vi "Find Broken VIs.vi"() -> ()   [LabVIEW 2016]
doc: "A wrapper engine for finding the list of broken VIs in a folder."
uses:
  <vilib>/Utility/error.llb/DialogType.ctl
  SLL Queued State Machine/Queue Driver/Create Queue.vi
  SLL Queued State Machine/Queue Driver/Enqueue an Item to Queue.vi
  SLL Queued State Machine/Queue Driver/Dequeue Queue.vi
  SLL Queued State Machine/Queue Driver/Enqueue N Items.vi
  SLL Queued State Machine/Queue Driver/Flush Queue.vi
  SLL Queued State Machine/Queue Driver/Release Queue.vi
  SLL Queued State Machine/SLL QSM.lvlib
  SLL Scripting/SLL Scripting.lvlib
panel:
  out "Number of VIs Broken":i32
  out "VIs Broken[]":path[](array[path])
  in  "Folder Path":path
  out "Status":string
  in  "Run":bool
  # "Find Broken VIs"
  # "Finds the list of broken VIs in a folder."
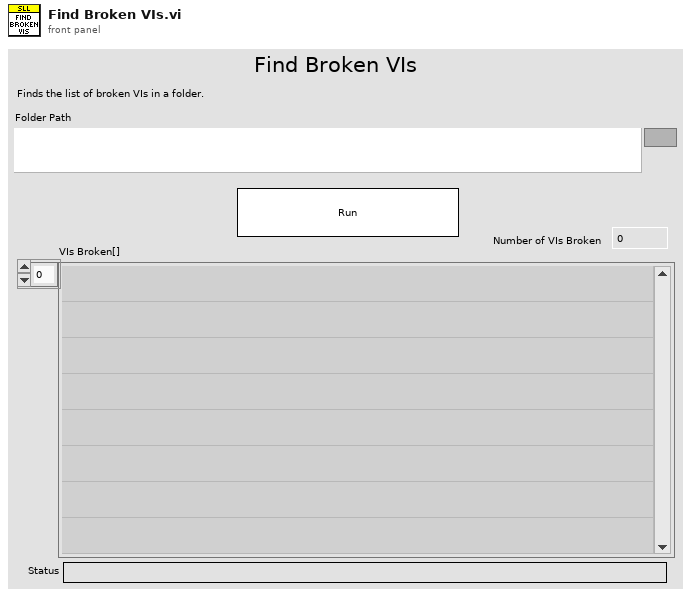
[diagram p1: front panel]
types:
  T1 = typedef "DialogType.ctl" = u16
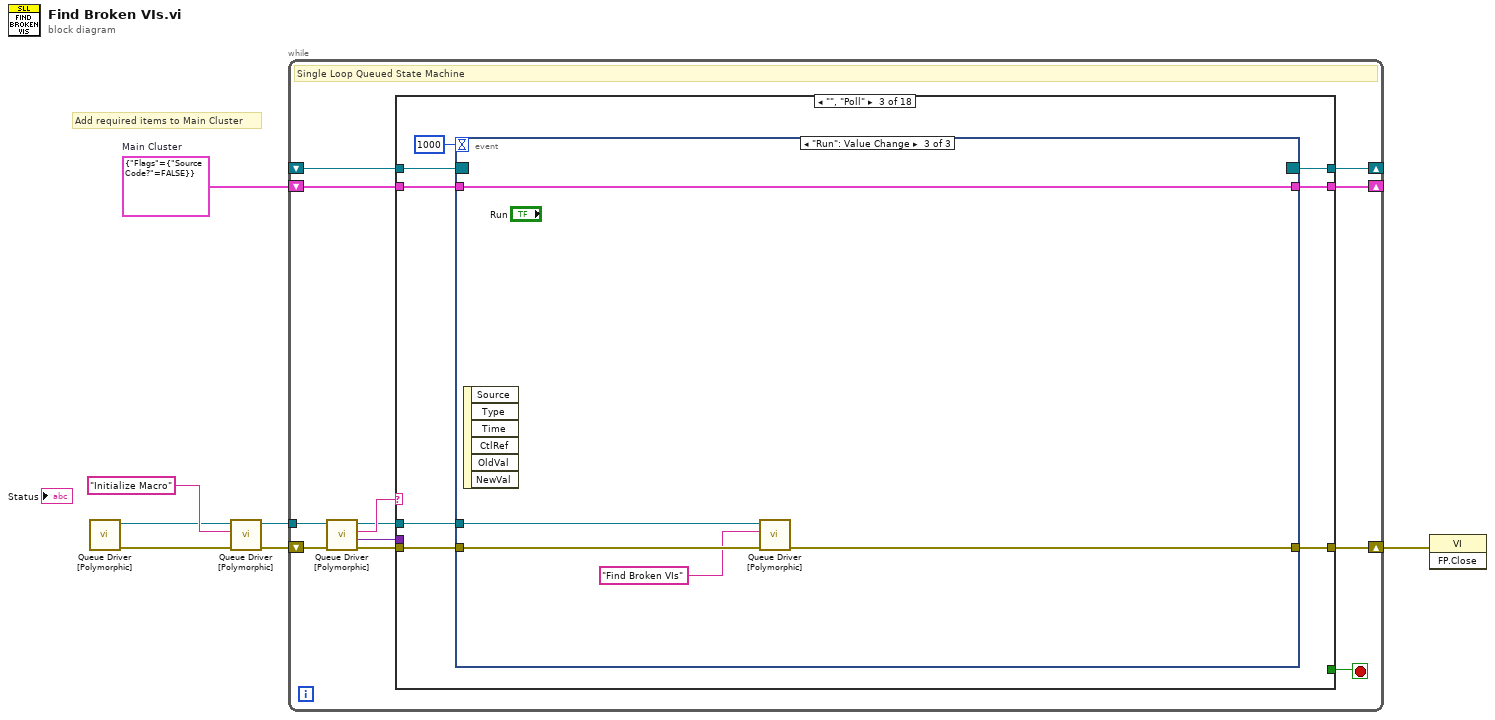
[diagram p0: block diagram]
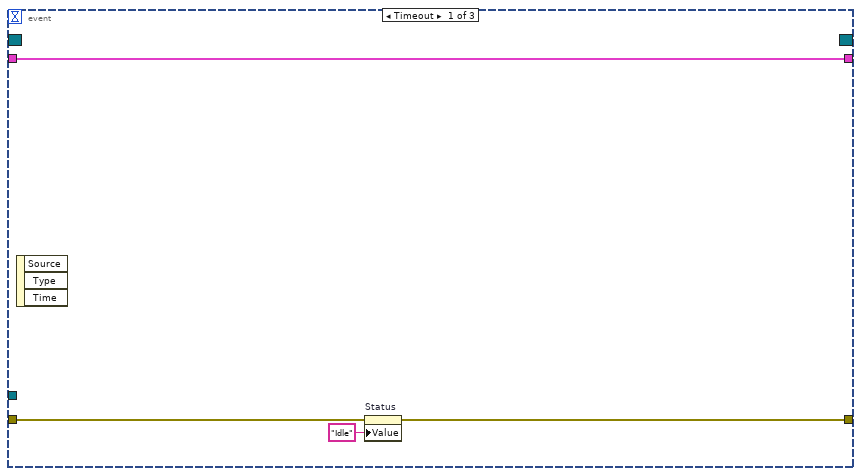
[diagram p4: hidden frame]
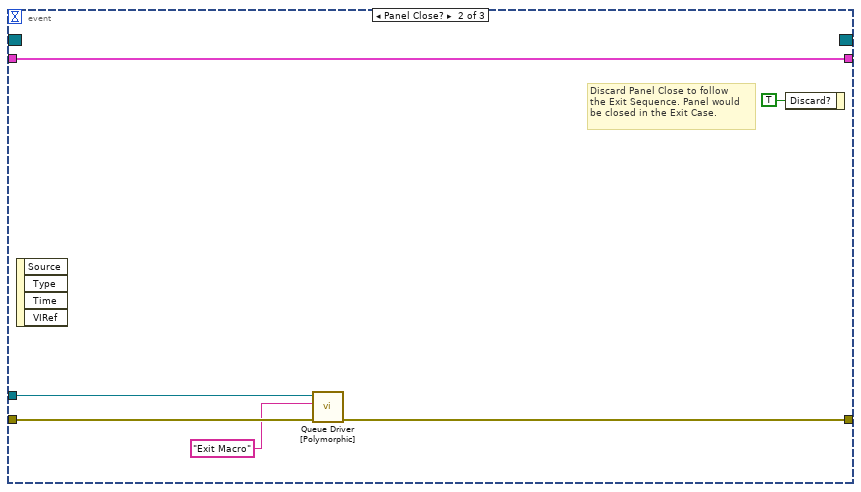
[diagram p5: hidden frame]
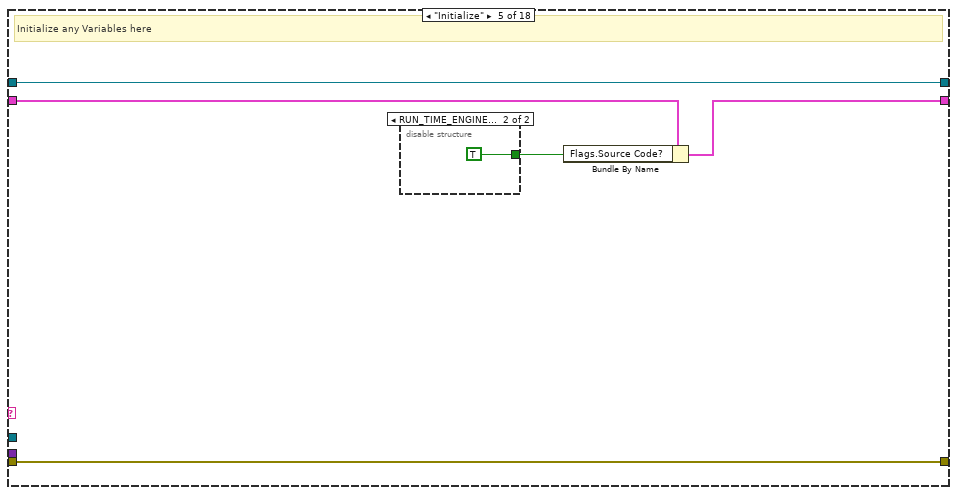
[diagram p7: hidden frame]
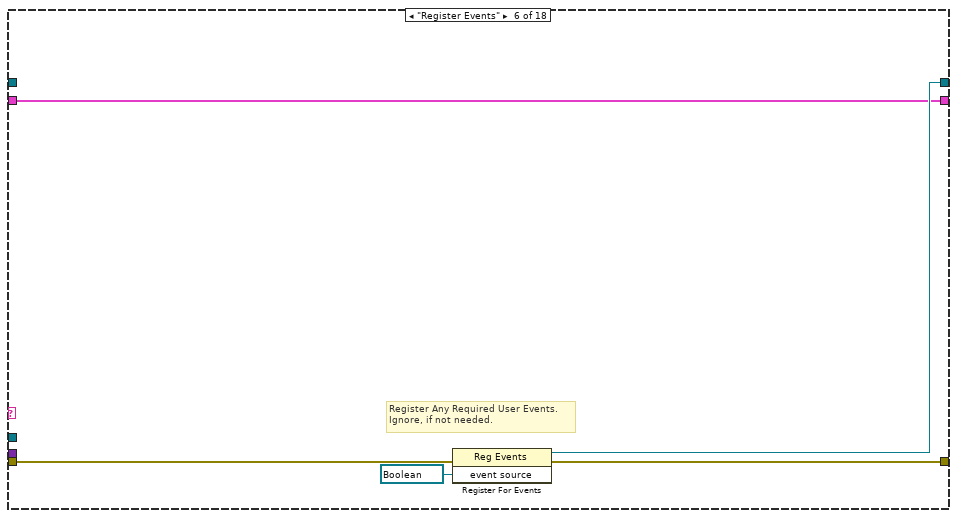
[diagram p9: hidden frame]
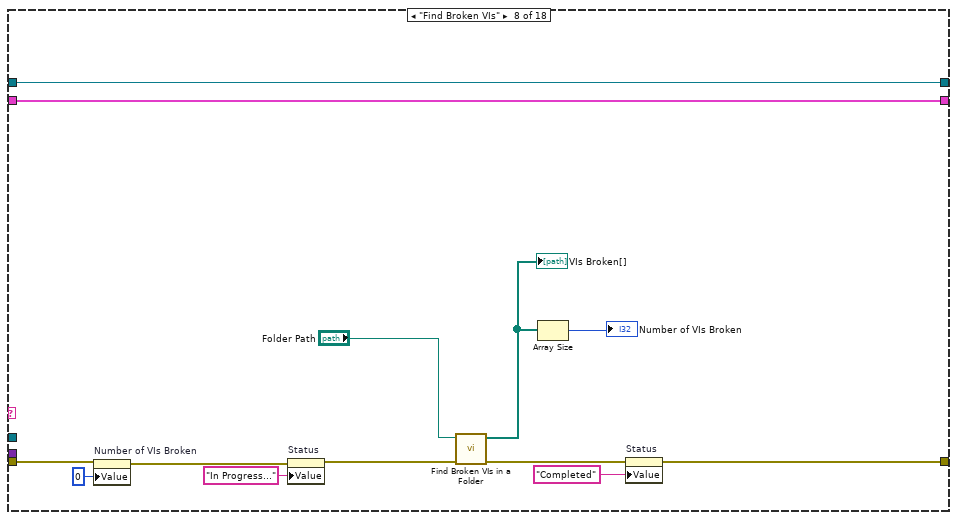
[diagram p11: hidden frame]
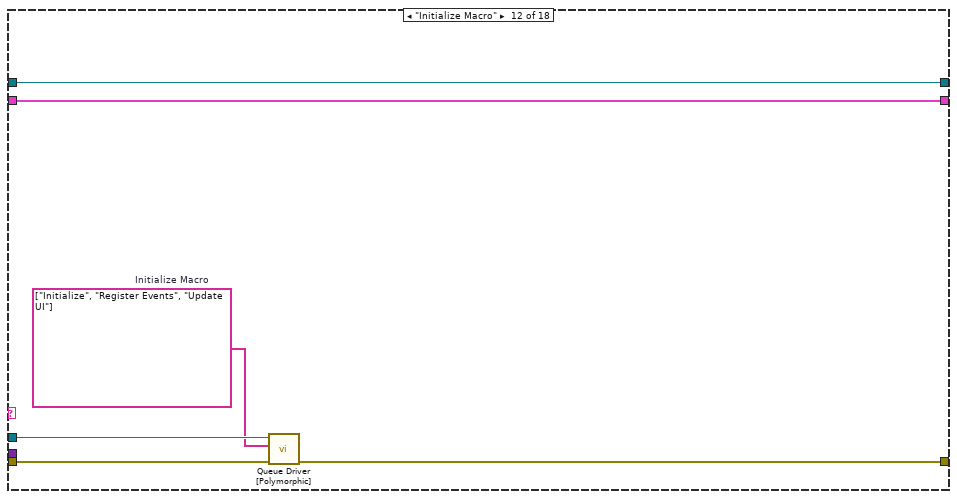
[diagram p15: hidden frame]
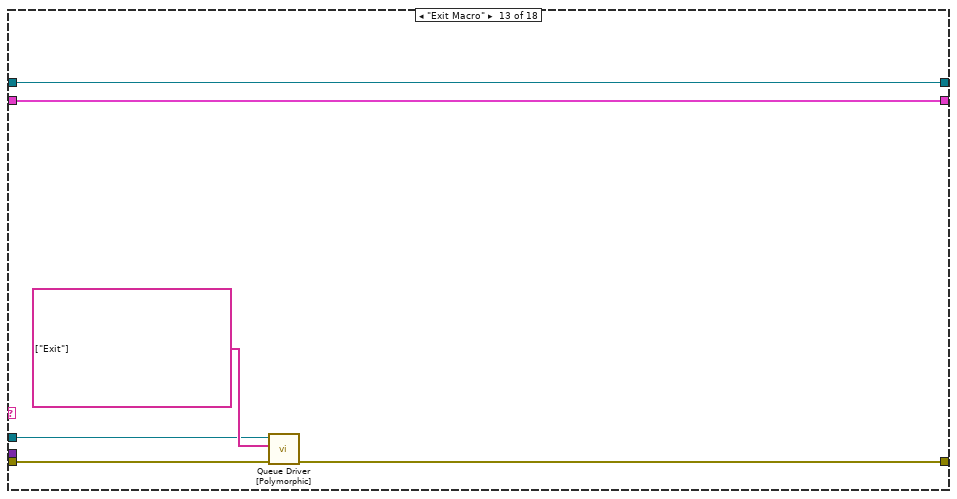
[diagram p16: hidden frame]
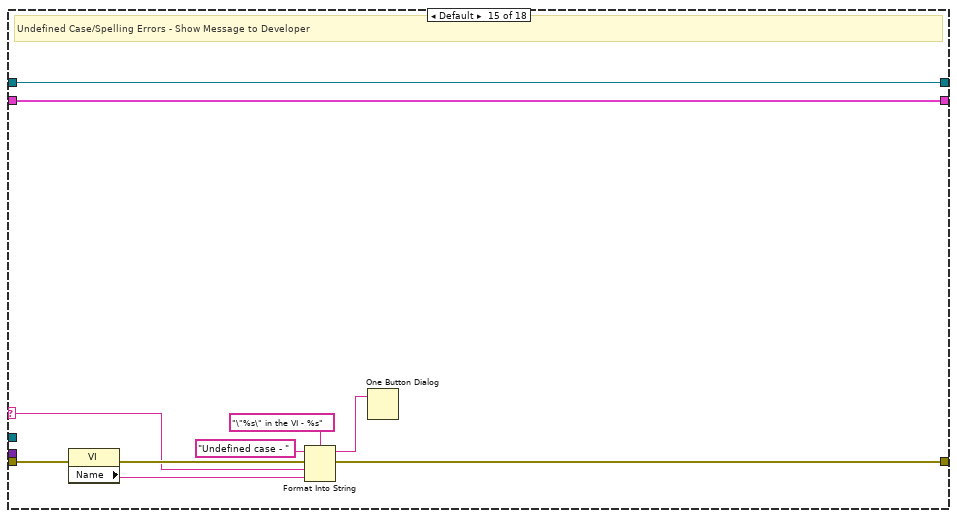
[diagram p18: hidden frame]
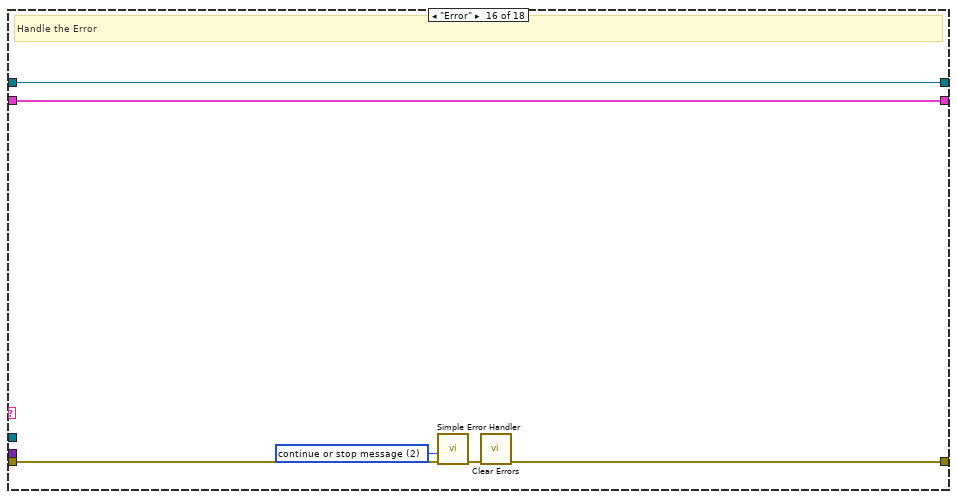
[diagram p19: hidden frame]
diagram:
  w5 = cluster{"Flags":cluster{"Source Code?":bool}} {"Flags"={"Source Code?"=FALSE}}  # Main Cluster
  # "Add required items to Main Cluster"
  n1 = call-poly "Queue Driver [Polymorphic].vi"() -> ("Error Out"=w7:errorcluster, "Queue Ref"=w3:refnum<queue>)  [unwired: 10 in]
  n2 = call-poly "Queue Driver [Polymorphic].vi"("Error In"=w7, "Item to Add"="Initialize Macro", "Queue Ref In"=w3) -> ("Error Out"=w6:errorcluster, "Queue Ref Out"=w2:refnum<queue>)  [unwired: 7 in]
  n3 = while "SLL Queued State Machine" {
    shift-right: [w17] -> w1
    shift-left: w6 -> [w19]
    shift-right: [w15] -> _
    shift-left: _ -> [w14]
    shift-right: [w13] -> _
    shift-left: w5 -> [w12]
    tunnel: w2 -> [w10]
    stop <- w16 stop-if-true
    # "Single Loop Queued State Machine"
    n4 = call-poly "Queue Driver [Polymorphic].vi"("Error In"=w19, "Queue Ref In"=w10) -> ("Error Out"=w18:errorcluster, "Data"=w8:variant, "Dequeue"=w11:string, "Queue Ref Out"=w9:refnum<queue>)  [unwired: 6 in]
    n5 = case "QSM Case Structure" shown="\"\", \"Poll\"" w11 {
      selector: w11 -> [_ _ _ _ _ _ _ _ _ _ _ _ _ _ w103 _ _ _]
      tunnel: w18 -> [w22 w25 w31 w51 w56 w62 w65 w68 w81 w84 w87 w91 w97 w102 w106 w118 w121 w134]
      tunnel: [w22 w25 w32 w51 w56 w61 w65 w73 w81 w84 w87 w90 w96 w102 w109 w116 w121 w130] -> w17
      tunnel: [_ _ _ _ _ _ _ _ _ _ _ _ _ _ _ _ _ TRUE] -> w16
      tunnel: [w21 w24 w30 w50 w55 w60 w64 w78 w80 w83 w86 w93 w99 w101 w112 w115 w120 w133] -> w15
      tunnel: w14 -> [w21 w24 w29 w50 w55 _ w64 w78 w80 w83 w86 w93 w99 w101 w112 w115 w120 w133]
      tunnel: [w20 w23 w27 w49 w52 w59 w63 w77 w79 w82 w85 w92 w98 w100 w111 w114 w119 w132] -> w13
      tunnel: w12 -> [w20 w23 w28 w49 w53 w59 w63 w77 w79 w82 w85 w92 w98 w100 w111 w114 w119 w132]
      tunnel: w9 -> [_ _ w26 _ _ _ _ _ _ _ _ w89 w94 _ _ _ _ w123]
      tunnel: w8 -> [_ _ _ _ _ _ _ _ _ _ _ _ _ _ _ _ _ _]
      frame "/--------------- Read Me -----------------/" {
        # "General Purpose Queue Based State Machine for Any Use Case (main application, module, pop up message etc)\n\nAdvantages:\n1. No Need to Pass Queue References between Queue Driver VIs.\n2. This template can be safely used in multiple parallel running modules without any issues.\n3. This template can also be safely used even in cases where the VI is configured to be a Clone, where multiple \ninstances of the VI could be executing concurrently.\n\nHow to Use:\n1. Add necessary items to the Main Cluster.\n2. Use the Polymorphic Queue Driver for doing any queue operations. There is no need to pass the queue driver\nreference, as the Queue Driver automatically infers the reference based on the VI instance from which it is called.\n3. Add any required user events in the \"Register Events\" case. Ignore if not needed.\n4. Use \"Sequences\" section for defining any list of state calls, which could be used in multiple places. \nEg: Initialize Sequence, might be needed if we need to any reinitialization."
      }
      frame "/------------------ Poll -------------------/" {
      }
      frame "", "Poll" {
        n6 = event shown="[2] \"Run\": Value Change" {
          selector: w29 -> [_ _ _]
          dyn-events: [_ _ _] -> w30
          timeout: 1000 -> [_ _ _]
          tunnel: [w34 w42 w47] -> w32
          tunnel: w31 -> [w35 w43 w48]
          tunnel: w28 -> [w37 w41 w46]
          tunnel: [w37 w41 w46] -> w27
          tunnel: w26 -> [_ w38 w44]
          event Timeout {
            n7 = event-data() -> ()  [unwired: 1 in, 3 out]
            n8 = property on="Status" class="Str"(error in=w35, "Value"="Idle" ("Status")) -> (error out=w34:errorcluster)  [unwired: 1 in, 1 out]
          }
          event Panel Close? {
            # "Discard Panel Close to follow\nthe Exit Sequence. Panel would\nbe closed in the Exit Case."
            n9 = event-data() -> ()  [unwired: 1 in, 4 out]
            n10 = call-poly "Queue Driver [Polymorphic].vi"("Error In"=w43, "Item to Add"="Exit Macro" ("Enqueue"), "Queue Ref In"=w38) -> ("Error Out"=w42:errorcluster)  [unwired: 7 in, 1 out]
            n11 = event-data("Discard?"=TRUE) -> ()  [unwired: 1 in, 1 out]
          }
          event "Run": Value Change {
            n12 = event-data() -> ()  [unwired: 1 in, 6 out]
            n13 = call-poly "Queue Driver [Polymorphic].vi"("Error In"=w48, "Item to Add"="Find Broken VIs" ("Enqueue"), "Queue Ref In"=w44) -> ("Error Out"=w47:errorcluster)  [unwired: 7 in, 1 out]
          }
        }
      }
      frame "/--------------- Initialize -----------------/" {
      }
      frame "Initialize" {
        # "Initialize any Variables here"
        n14 = disable-structure shown="RUN_TIME_ENGINE==False" {
          disable-tunnel: [_ TRUE] -> w54
          frame condition #0 {
          }
          frame condition #1 (active) {
          }
        }
        n15 = Bundle By Name(cluster=w53, "Flags.Source Code?"=w54) -> (w52:cluster{"Flags":cluster{"Source Code?":bool}})
      }
      frame "Register Events" {
        # "Register Any Required User Events. \nIgnore, if not needed."
        n16 = register-events(error in=w62, refnum<vi> refnum ("event source")) -> (reference out=w60:refnum<event-registration>, error out=w61:errorcluster)  [unwired: 1 in]
      }
      frame "/---------- Custom Case Splitter ----------/" {
      }
      frame "Find Broken VIs" {
        n17 = property on="Number of VIs Broken" class="DigNum (strict)"(error in=w68, "Value"=0 ("Number of VIs Modified")) -> (error out=w67:errorcluster)  [unwired: 1 in, 1 out]
        n18 = property on="Status" class="Str"(error in=w67, "Value"="In Progress..." ("Status")) -> (error out=w76:errorcluster)  [unwired: 1 in, 1 out]
        n19 = call "Find Broken VIs in a Folder.vi"("error in (no error)"=w76, "Directory Path"="Folder Path") -> ("error out"=w74:errorcluster, "Broken VIs"=w70:path[])  [unwired: 8 in]
        "VIs Broken[]" <- w70
        n20 = Array Size(array=w70) -> (size(s)=→"Number of VIs Broken":i32)
        n21 = property on="Status" class="Str"(error in=w74, "Value"="Completed" ("Status")) -> (error out=w73:errorcluster)  [unwired: 1 in, 1 out]
      }
      frame "/-------------- User Interface --------------/" {
        # "Duplicate this case to create additional case splitters for readability"
      }
      frame "Update UI" {
        # "Update Front Panel Controls in this Case"
      }
      frame "/----------------- Macros -----------------/" {
      }
      frame "Initialize Macro" {
        w88 = string[] ["Initialize", "Register Events", "Update UI"]  # Initialize Macro
        n22 = call-poly "Queue Driver [Polymorphic].vi"("Error In"=w91, "Enqueue N"=w88, "Queue Ref In"=w89) -> ("Error Out"=w90:errorcluster)  [unwired: 7 in, 1 out]
      }
      frame "Exit Macro" {
        n23 = call-poly "Queue Driver [Polymorphic].vi"("Error In"=w97, "Enqueue N"=string[] ["Exit"], "Queue Ref In"=w94) -> ("Error Out"=w96:errorcluster)  [unwired: 7 in, 1 out]
      }
      frame "/-------------- Error Handler--------------/" {
      }
      frame Default {
        # "Undefined Case/Spelling Errors - Show Message to Developer"
        n24 = property class="VI"(error in=w106) -> (error out=w105:errorcluster, "Name"=w104:string)  [unwired: 1 in, 1 out]
        n25 = Format Into String(format string="\"%s\" in the VI - %s" ("message"), initial string="Undefined case - ", error in=w105, w103, w104) -> (resulting string=w107:string, error out=w109:errorcluster)
        n26 = One Button Dialog(message=w107) -> ()  [unwired: 1 in, 1 out]
      }
      frame "Error" {
        w113 = T1 2 items=["no dialog", "OK message", "continue or stop message", "OK message + warnings", "continue/stop + warnings"] ("type of dialog (OK msg:1)")
        # "Handle the Error"
        n27 = call <vilib>:"Simple Error Handler.vi"("type of dialog (OK msg:1)"=w113, "error in (no error)"=w118) -> ("error out"=w117:errorcluster)  [unwired: 3 in, 4 out]
        n28 = call <vilib>:"Clear Errors.vi"("error in (no error)"=w117) -> ("error out"=w116:errorcluster)  [unwired: 5 in, 1 out]
      }
      frame "/------------------- Exit --------------------/" {
      }
      frame "Exit" {
        n29 = call-poly "Queue Driver [Polymorphic].vi"("Error In"=w134, "Queue Ref In"=w123) -> ("Error Out"=w135:errorcluster, "Queue Ref Out"=w122:refnum<queue>)  [unwired: 7 in, 1 out]
        n30 = Unbundle By Name(w132) -> ("Flags.Source Code?"=w125:bool)
        n31 = call-poly "Queue Driver [Polymorphic].vi"("Error In"=w135, "Queue Ref In"=w122) -> ("Error Out"=w131:errorcluster)  [unwired: 9 in]
        n32 = Call Chain() -> (call chain=w129:string[])
        n33 = Array Size(array=w129) -> (size(s)=w128:i32)
        n34 = Equal?(x=w128, y=1) -> (x = y?=w126:bool)
        n35 = And(x=w125, y=w126) -> (x .and. y?=w124:bool)
        n36 = case "Skip Panel Close when in Source\nCode and is the top most caller" shown="True" w124 {
          tunnel: w131 -> [w138 w140]
          tunnel: [w139 w140] -> w130
          frame False {
            # "Close Panel"
            n37 = invoke class="VI" method="FP.Close"() -> (error out=w137:errorcluster)  [unwired: 3 in, 2 out]
            n38 = Merge Errors(w138, w137) -> (w139:errorcluster)
          }
          frame True {
            # "Do Not Close Panel"
          }
        }
      }
    }
  }
  n39 = invoke class="VI" method="FP.Close"(error in=w1) -> ()  [unwired: 2 in, 3 out]
